vi "Get Active Alarms V.vi"(8 "error in (no error)":errorcluster, 11 "alarmFieldStruct":T1) -> (0 "error out":errorcluster, 2 "function return":i16, 3 "alarmFieldStruct out":T1)   [LabVIEW 2009, in "VantagePro.lvlib"]
doc: "DllAccess short int _stdcall GetActiveAlarms_V( ActiveAlarmFields &alarmFieldStruct );"
uses:
  VantagePro.lvlib
  <userlib>/VantagePro/VantagePro.dll
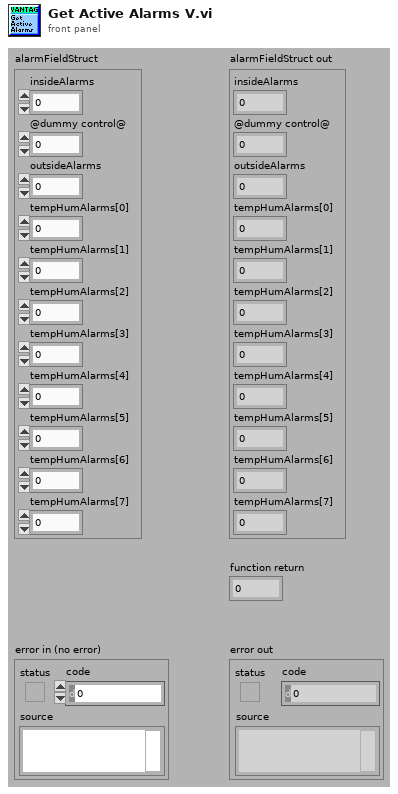
[diagram p1: front panel]
types:
  T1 = cluster{"insideAlarms":u8, "@dummy control@":i8, "outsideAlarms":u16, "tempHumAlarms[0]":u8, "tempHumAlarms[1]":u8, "tempHumAlarms[2]":u8, "tempHumAlarms[3]":u8, "tempHumAlarms[4]":u8, "tempHumAlarms[5]":u8, "tempHumAlarms[6]":u8, "tempHumAlarms[7]":u8}
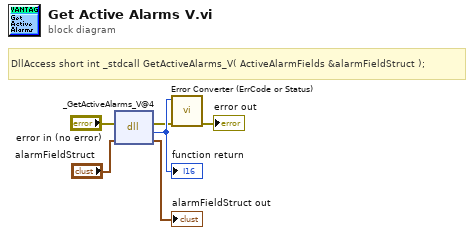
[diagram p0: block diagram]
diagram:
  # "DllAccess short int _stdcall GetActiveAlarms_V( ActiveAlarmFields &alarmFieldStruct );"
  n1 = dll-call lib="C:/Program Files/National Instruments/LabVIEW 2010/user.lib/VantagePro/VantagePro.*" fn="_GetActiveAlarms_V@4"(error in="error in (no error)", "alarmFieldStruct"="alarmFieldStruct") -> (error out=w2:errorcluster, w6:i16, "alarmFieldStruct"=→"alarmFieldStruct out":T1)  [unwired: 2 in, 1 out]
  "function return" <- w6
  n2 = call "Error Converter (ErrCode or Status).vi"("error in (no error)"=w2, "error code"=w6) -> ("error out"=→"error out":errorcluster)  [unwired: 9 in]
